vi "Read Data.vi"(8 "error in":errorcluster, 11 "CutomOOB_Tx in":refnum<class "CIFCustomOOB_Tx.lvclass">) -> (0 "error out":errorcluster, 2 "Data":cluster{"Numeric":i32}, 3 "CutomOOB_Tx out":refnum<class "CIFCustomOOB_Tx.lvclass">)   [LabVIEW 2021, in "CIFCustomOOB_Tx.lvclass"]
uses:
  CIFCustomOOB_Tx.lvclass
  CIFCustomOOB_Tx.lvclass/CIFCustomOOB_Tx.ctl
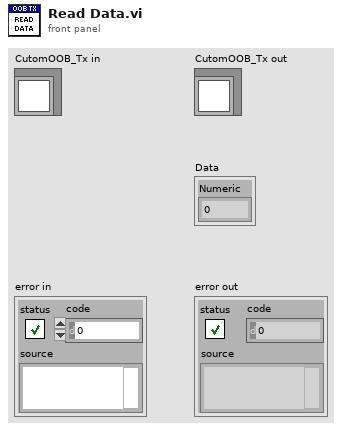
[diagram p1: front panel]
types:
  T1 = typedef "CIFCustomOOB_Tx.lvclass/Payload.ctl" = cluster{"Data":cluster{"Numeric":i32}}
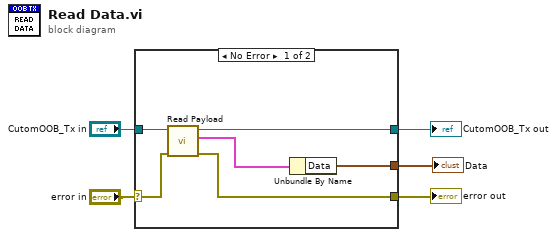
[diagram p0: block diagram]
diagram:
  n1 = case shown="No Error" "error in" {
    selector: "error in" -> [w9 w13]
    tunnel: [w8 w13] -> w5
    tunnel: [w10 w12] -> w4
    tunnel: "CutomOOB_Tx in" -> [w11 w12]
    tunnel: [w6 _] -> w1
    frame No Error {
      n2 = call "Read Payload.vi"("error in"=w9, "CutomOOB_Tx in"=w11) -> ("error out"=w8:errorcluster, "data"=w7:T1, "CutomOOB_Tx out"=w10:refnum<class "CIFCustomOOB_Tx.lvclass">)  [unwired: 7 in]
      n3 = Unbundle By Name(w7) -> ("Data"=w6:cluster{"Numeric":i32})
    }
    frame Error {
    }
  }
  "error out" <- w5
  "CutomOOB_Tx out" <- w4
  "Data" <- w1
